vi "Wire Measurement Wrapper Alone.vi"(0 "vi reference":refnum<vi>, 5 "sub vi in":refnum<vi>[](array[refnum]), 7 "terminal":refnum<vi>, 11 "error in":errorcluster) -> (15 "error out":errorcluster)   [LabVIEW 2021, in "Converter.lvlib"]
uses:
  Converter.lvlib
  Converter Reusables/Converter Reusables.lvlib
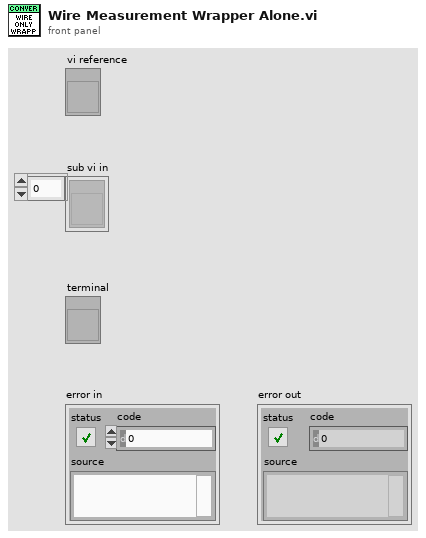
[diagram p1: front panel]
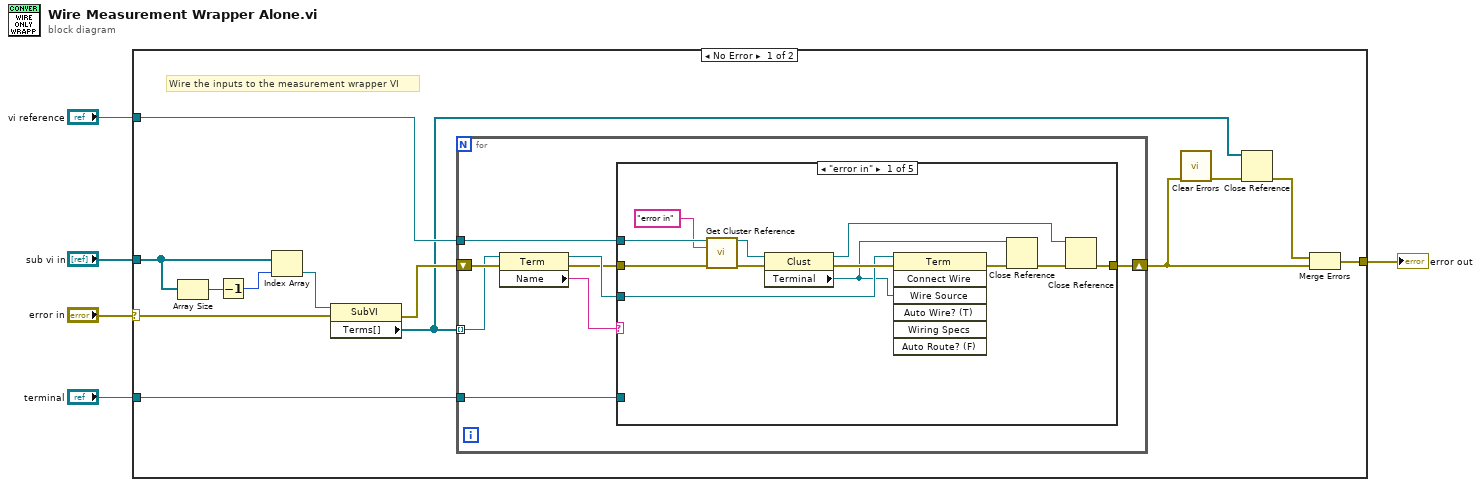
[diagram p0: block diagram]
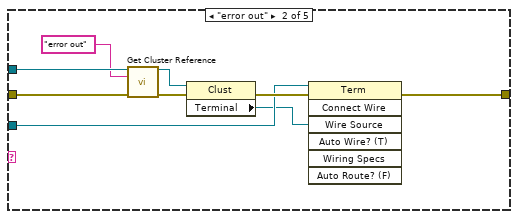
[diagram p2: hidden frame]
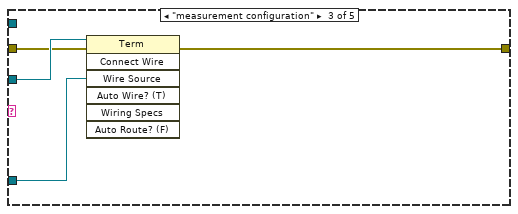
[diagram p3: hidden frame]
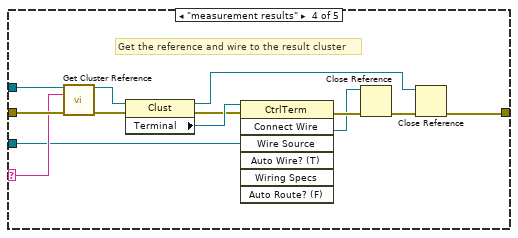
[diagram p4: hidden frame]
diagram:
  n1 = case shown="No Error" "error in" {
    selector: "error in" -> [w15 w66]
    tunnel: "vi reference" -> [w17 _]
    tunnel: [w12 w66] -> w1
    tunnel: "sub vi in" -> [w7 _]
    tunnel: "terminal" -> [w11 _]
    frame No Error {
      # "Wire the inputs to the measurement wrapper VI"
      n2 = Array Size(array=w7) -> (size(s)=w14:i32)
      n3 = Decrement(x=w14) -> (x-1=w8:i32)
      n4 = Index Array(array=w7, index=w8) -> (element=w18:refnum<vi>)
      n5 = property class="SubVI"(reference=w18, error in=w15) -> (error out=w13:errorcluster, "Terms[]"=w10:refnum<vi>[])  [unwired: 1 out]
      n6 = for {
        tunnel: w10 -> [w25] mode=indexing
        tunnel: w11 -> [w24]
        tunnel: w17 -> [w23]
        shift-right: [w22] -> w6
        shift-left: w13 -> [w26]
        n7 = property class="Term"(reference=w25, error in=w26) -> (reference out=w20:refnum<vi>, error out=w19:errorcluster, "Name"=w21:string)
        n8 = case shown="\"error in\"" w21 {
          selector: w21 -> [_ _ _ w63 _]
          tunnel: w20 -> [w28 w43 w51 w52 _]
          tunnel: w24 -> [_ _ w49 _ _]
          tunnel: w19 -> [w32 w47 w50 w64 w65]
          tunnel: [w34 w46 w48 w55 w65] -> w22
          tunnel: w23 -> [w31 w42 _ w62 _]
          frame "error in" {
            n9 = call "Get Cluster Reference.vi"("vi in"=w31, "name/order"="error in", "error in"=w32) -> ("cluster out"=w29:refnum<vi>, "error out"=w37:errorcluster)  [unwired: 11 in]
            n10 = property class="Clust"(reference=w29, error in=w37) -> (reference out=w33:refnum<vi>, error out=w36:errorcluster, "Terminal"=w27:refnum<vi>)
            n11 = invoke class="Term" method="Connect Wire"(reference=w28, error in=w36, "Wire Source"=w27) -> (error out=w38:errorcluster)  [unwired: 4 in, 6 out]
            n12 = Close Reference(reference=w27, error in (no error)=w38) -> (error out=w35:errorcluster)
            n13 = Close Reference(reference=w33, error in (no error)=w35) -> (error out=w34:errorcluster)
          }
          frame "error out" {
            n14 = call "Get Cluster Reference.vi"("vi in"=w42, "name/order"="error out", "error in"=w47) -> ("cluster out"=w41:refnum<vi>, "error out"=w45:errorcluster)  [unwired: 11 in]
            n15 = property class="Clust"(reference=w41, error in=w45) -> (error out=w44:errorcluster, "Terminal"=w40:refnum<vi>)  [unwired: 1 out]
            n16 = invoke class="Term" method="Connect Wire"(reference=w43, error in=w44, "Wire Source"=w40) -> (error out=w46:errorcluster)  [unwired: 4 in, 6 out]
          }
          frame "measurement configuration" {
            n17 = invoke class="Term" method="Connect Wire"(reference=w51, error in=w50, "Wire Source"=w49) -> (error out=w48:errorcluster)  [unwired: 4 in, 6 out]
          }
          frame "measurement results" {
            # "Get the reference and wire to the result cluster"
            n18 = call "Get Cluster Reference.vi"("vi in"=w62, "name/order"=w63, "error in"=w64) -> ("cluster out"=w56:refnum<vi>, "error out"=w61:errorcluster)  [unwired: 11 in]
            n19 = property class="Clust"(reference=w56, error in=w61) -> (reference out=w53:refnum<vi>, error out=w59:errorcluster, "Terminal"=w60:refnum<vi>)
            n20 = invoke class="CtrlTerm" method="Connect Wire"(reference=w60, error in=w59, "Wire Source"=w52) -> (reference out=w54:refnum<vi>, error out=w58:errorcluster)  [unwired: 4 in, 5 out]
            n21 = Close Reference(reference=w54, error in (no error)=w58) -> (error out=w57:errorcluster)
            n22 = Close Reference(reference=w53, error in (no error)=w57) -> (error out=w55:errorcluster)
          }
          frame Default {
          }
        }
      }
      n23 = call <vilib>:"Clear Errors.vi"("error in (no error)"=w6) -> ("error out"=w16:errorcluster)  [unwired: 5 in, 1 out]
      n24 = Close Reference(reference=w10, error in (no error)=w16) -> (error out=w9:errorcluster)
      n25 = Merge Errors(w9, w6) -> (w12:errorcluster)
    }
    frame Error {
    }
  }
  "error out" <- w1
